vi "Verify Errors Array.vi"(8 "error in (no error)":errorcluster, 11 "Simulated_CCD_Camera in":refnum<class "Sim_Ixon_Ultra.lvclass">) -> (0 "error out":errorcluster, 3 "Simulated_CCD_Camera out":refnum<class "Sim_Ixon_Ultra.lvclass">)   [LabVIEW 2018, in "Sim_Ixon_Ultra.lvclass"]
doc: "Verify the erro array.\n\nThis function returns true if there is any element of the array with an error. Otherwise, it returns false"
uses:
  Sim_Ixon_Ultra.lvclass
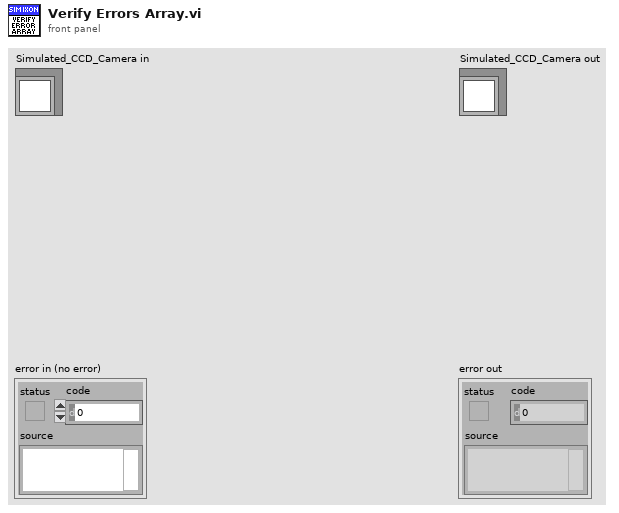
[diagram p1: front panel]
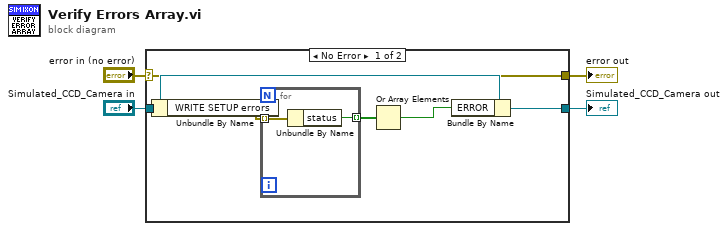
[diagram p0: block diagram]
diagram:
  n1 = case shown="No Error" "error in (no error)" {
    selector: "error in (no error)" -> [w7 w14]
    tunnel: [w7 w14] -> w3
    tunnel: [w6 w13] -> w1
    tunnel: "Simulated_CCD_Camera in" -> [w8 w13]
    frame No Error {
      n2 = Unbundle By Name(w8) -> ("WRITE SETUP errors"=w10:errorcluster[])
      n3 = for {
        tunnel: w10 -> [w12] mode=indexing
        tunnel: [w11] -> w9 mode=indexing
        n4 = Unbundle By Name(w12) -> ("status"=w11:bool)
      }
      n5 = Or Array Elements(Boolean array=w9) -> (logical OR=w5:bool)
      n6 = Bundle By Name(cluster=w8, "ERROR"=w5) -> (w6:refnum<class "Sim_Ixon_Ultra.lvclass">)
    }
    frame Error {
    }
  }
  "error out" <- w3
  "Simulated_CCD_Camera out" <- w1
